vi "PicohrdlGetMinMaxAdcCounts.vi"(8 "error in (no error)":errorcluster, 9 "channel":i16=-1, 11 "handle in":i16) -> (0 "error out":errorcluster, 1 "minAdc":i32, 2 "maxAdc":i32, 3 "handle out":i16)   [LabVIEW 2010]
doc: "Calls HRDLGetMinMaxAdcCounts()s"
uses:
  PicoHRDL.dll
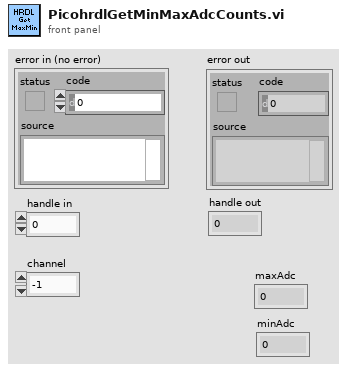
[diagram p1: front panel]
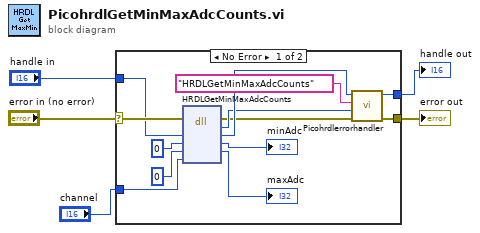
[diagram p0: block diagram]
diagram:
  n1 = case shown="No Error" "error in (no error)" {
    selector: "error in (no error)" -> [w12 w19]
    tunnel: "handle in" -> [w11 w20]
    tunnel: [w9 w20] -> w5
    tunnel: [w10 w19] -> w4
    tunnel: "channel" -> [w7 _]
    frame No Error {
      n2 = dll-call lib="PicoHRDL.dll" fn="HRDLGetMinMaxAdcCounts"(error in=w12, "handle"=w11, "minAdc"=0 ("maxAdc"), "maxAdc"=0, "channel"=w7) -> (error out=w15:errorcluster, "return type"=w16:i32, "handle"=w18:i16, "minAdc"=→"minAdc":i32, "maxAdc"=→"maxAdc":i32)  [unwired: 3 in, 1 out]
      n3 = call "Picohrdlerrorhandler.vi"("Handle in"=w18, "API function"="HRDLGetMinMaxAdcCounts", "Return"=w16, "error in (no error)"=w15) -> ("Handle out"=w9:i16, "error out"=w10:errorcluster)  [unwired: 5 in]
    }
    frame Error {
    }
  }
  "error out" <- w4
  "handle out" <- w5
